vi "Monitor Data Changed.vi"(8 "error in (no error)":errorcluster, 9 "Changed Actor's Q":refnum<class "Message Enqueuer.lvclass">, 10 "Monitor Data":refnum<class "Monitor Data.lvclass">, 11 "Actor Monitor New in":refnum<class "Actor Monitor.lvclass">) -> (0 "error out":errorcluster, 3 "Actor Monitor New out":refnum<class "Actor Monitor.lvclass">)   [LabVIEW 2017, in "MGI-Monitored Actor Core.lvlib" / "Actor Monitor.lvclass"]
doc: "Called any time the monitor data is changed. Use the \"Changed Actor's Q\" to determine what actor has changed.\n\nCopyright: MGI 2016\nAuthor: Derek Trepanier"
uses:
  Actor Monitor.lvclass
  Monitor Data/Monitor Data.lvclass
  <vilib>/ActorFramework/Message Enqueuer/Message Enqueuer.lvclass
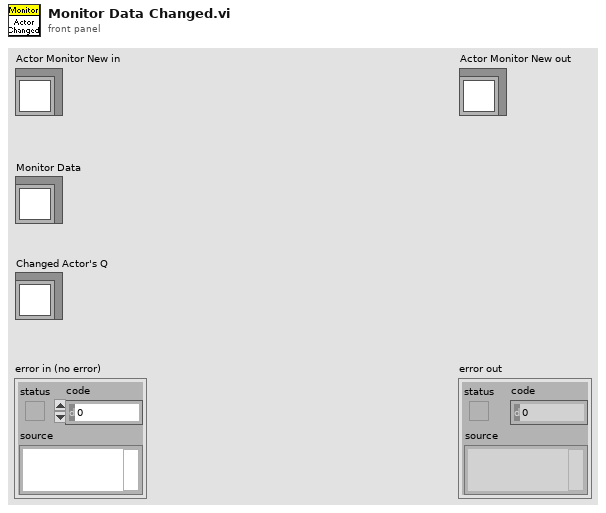
[diagram p1: front panel]
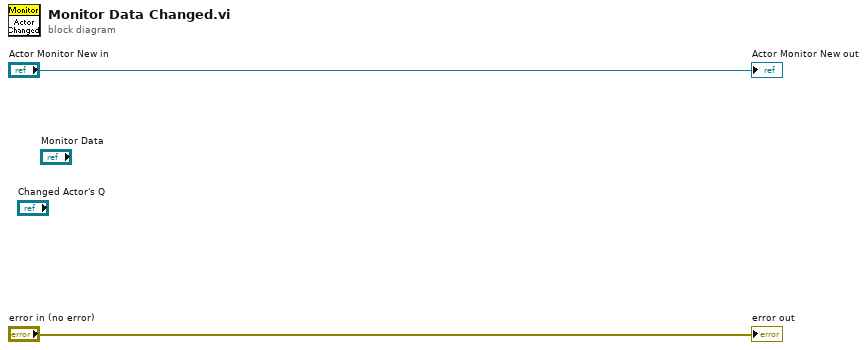
[diagram p0: block diagram]
diagram:
  "error out" <- "error in (no error)"
  "Actor Monitor New out" <- "Actor Monitor New in"
